vi "weightedAccumulator.vi"(7 "reset":bool, 8 "inputValid":bool, 10 "weight":fxp<+,16,0>, 11 "input":i16) -> (0 "outputValid":bool, 3 "weightedSum":fxp<+/-,54,34>)   [LabVIEW 2016]
uses:
  <vilib>/rvi/FXPMathLib/FxpInterpret/XNode/nifxpmath_Interpret.xnode
  <vilib>/rvi/FXPMathLib/FxpMul/XNode/nifxpmath_Multiplier.xnode
  <vilib>/rvi/FXPMathLib/FxpAdd/XNode/nifxpmath_Add.xnode
  <vilib>/rvi/FXPMathLib/sim/FxpSim.dll
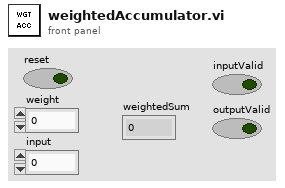
[diagram p1: front panel]
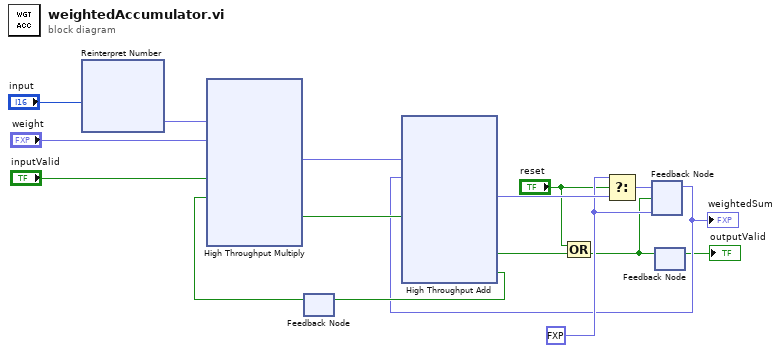
[diagram p0: block diagram]
diagram:
  w10 = fxp<+/-,53,33> 0.0 ("x+y")
  n1 = xnode "Reinterpret Number"("x"="input") -> ("y"=w12:fxp<+/-,16,16>)
  n2 = feedback #1() -> (w7:bool)  [unwired: 1 in]
  n3 = xnode ("High Throughput Multiply")("x"=w12, "y"="weight", "input valid"="inputValid", "ready for output (T)"=w7) -> ("x*y"=w14:fxp<+/-,32,16>, "output valid"=w9:bool)  [unwired: 1 out]
  n4 = feedback #2(w10) -> (w6:fxp<+/-,53,33>)
  "weightedSum" <- w6
  n5 = xnode ("High Throughput Add")("x"=w14, "y"=w6, "input valid"=w9) -> ("x+y"=w15:fxp<+/-,52,32>, "output valid"=w4:bool, "ready for input"=w8:bool)  [unwired: 1 in]
  n6 = feedback-in #1(w8) -> ()
  n7 = Compound Arithmetic op=OR("reset", w4) -> (w2:bool)
  n8 = Select(t=w10, s="reset", f=w15) -> (s? t:f=w11:fxp<+/-,53,33>)
  n9 = feedback-in #2(w11, w2) -> ()
  n10 = feedback-in #3(w2) -> ()
  n11 = feedback #3() -> (→"outputValid":bool)  [unwired: 1 in]
